vi "Write Device ID Type.vi"(8 "error in (no error)":errorcluster, 10 "device ID type":u8(ring)=1 items=["None"=0, "Basic Stream"=1, "Regular Stream"=2, "Extended Stream"=3, "Basic Stream/Individual"=129, "Regular Stream/Individual"=130, "Extended Stream/Individual"=131], 11 "device data model in":refnum<class "Standard Data Model.lvclass">) -> (0 "error out":errorcluster, 3 "device data model out":refnum<class "Standard Data Model.lvclass">)   [LabVIEW 2018, in "SubVIs.lvlib" / "Standard Data Model.lvclass"]
doc: "Writes the value of the device ID."
uses:
  Standard Data Model.lvclass
  Standard Data Model.lvclass/Standard Data Model.ctl
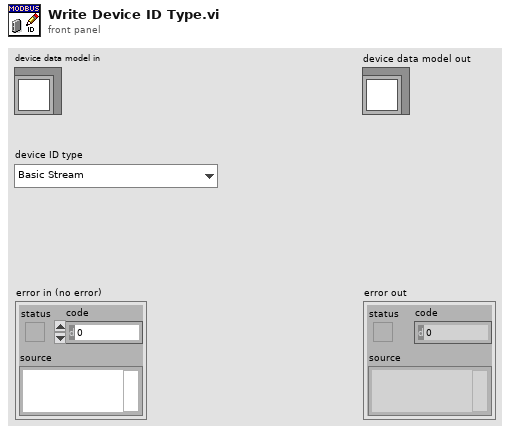
[diagram p1: front panel]
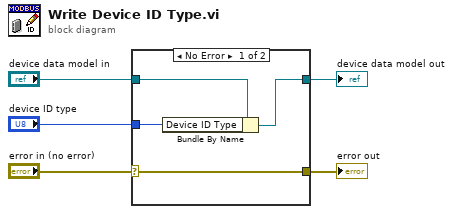
[diagram p0: block diagram]
diagram:
  n1 = case shown="No Error" "error in (no error)" {
    selector: "error in (no error)" -> [w6 w10]
    tunnel: "device data model in" -> [w9 w11]
    tunnel: [w8 w11] -> w4
    tunnel: "device ID type" -> [w7 _]
    tunnel: [w6 w10] -> w1
    frame No Error {
      n2 = Bundle By Name(cluster=w9, "Device ID Type"=w7) -> (w8:refnum<class "Standard Data Model.lvclass">)
    }
    frame Error {
    }
  }
  "error out" <- w1
  "device data model out" <- w4
